vi "elevatorStatesLogic.vi"(9 "oldState":T1, 10 "newState":T1, 11 "timer":i32) -> (0 "State":T1, 1 "manual?":bool, 2 "Numeric":i32, 3 "elevatorActive":bool)   [LabVIEW 2014]
uses:
  ElevatorStates.ctl
  Global Data!!!.vi
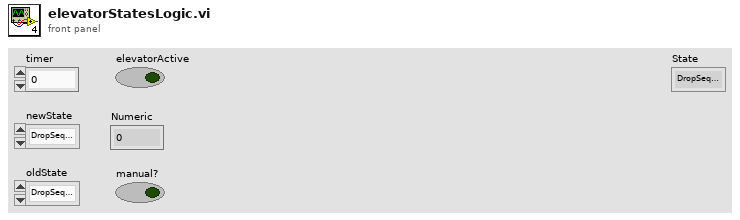
[diagram p1: front panel]
types:
  T1 = typedef "ElevatorStates.ctl" = enum16{"DropSequence", "Reset", "Drop1Stage", "2StageEngage", "Lift1Stage", "1StageEngage", "Rest", "InterruptedLift", "Manual", "Auto2Man", "Initialize", "FeederMode"}
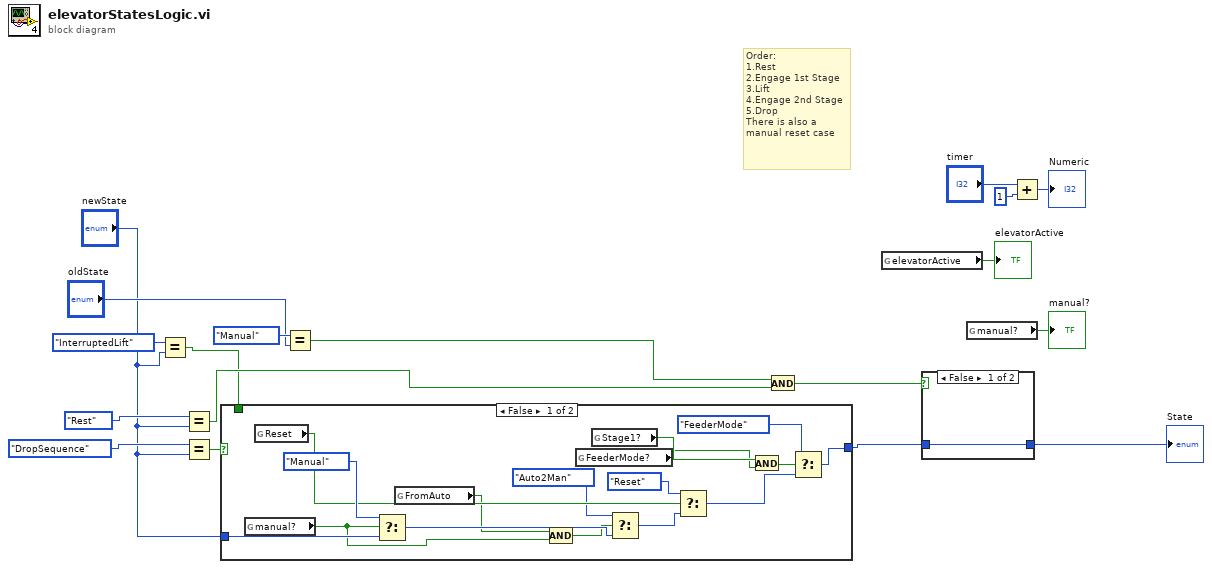
[diagram p0: block diagram]
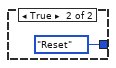
[diagram p2: hidden frame]
diagram:
  # "Order:\n1.Rest\n2.Engage 1st Stage\n3.Lift\n4.Engage 2nd Stage\n5.Drop\nThere is also a \nmanual reset case"
  n1 = Equal?(x=ElevatorStates."InterruptedLift", y="newState") -> (x = y?=w2:bool)
  n2 = Equal?(x=ElevatorStates."Rest", y="newState") -> (x = y?=w7:bool)
  n3 = Equal?(x=ElevatorStates."DropSequence", y="newState") -> (x = y?=w15:bool)
  n4 = case shown="False" w15 {
    tunnel: [w23 w35] -> w6
    tunnel: "newState" -> [w31 w35]
    tunnel: w2 -> [_ _]
    frame False {
      n5 = global read "Global Data!!!.vi" "manual?"() -> (w26:bool)
      n6 = global read "Global Data!!!.vi" "Reset"() -> (w33:bool)
      n7 = Select(t=ElevatorStates."Manual" ("Enum"), s=w26, f=w31) -> (s? t:f=w29:T1)
      n8 = global read "Global Data!!!.vi" "FromAuto"() -> (w25:bool)
      n9 = Compound Arithmetic op=AND(w25, w26) -> (w27:bool)
      n10 = global read "Global Data!!!.vi" "FeederMode?"() -> (w19:bool)
      n11 = global read "Global Data!!!.vi" "Stage1?"() -> (w20:bool)
      n12 = Select(t=ElevatorStates."Auto2Man", s=w27, f=w29) -> (s? t:f=w30:T1)
      n13 = Select(t=ElevatorStates."Reset" ("Enum"), s=w33, f=w30) -> (s? t:f=w24:T1)
      n14 = And(x=w20, y=w19) -> (x .and. y?=w21:bool)
      n15 = Select(t=ElevatorStates."FeederMode", s=w21, f=w24) -> (s? t:f=w23:T1)
    }
    frame True {
    }
  }
  n16 = Equal?(x=ElevatorStates."Manual", y="oldState") -> (x = y?=w9:bool)
  n17 = And(x=w9, y=w7) -> (x .and. y?=w10:bool)
  n18 = global read "Global Data!!!.vi" "elevatorActive"() -> (→"elevatorActive":bool)
  n19 = case shown="False" w10 {
    tunnel: w6 -> [w36 _]
    tunnel: [w36 ElevatorStates."Reset" ("newState")] -> w1
    frame False {
    }
    frame True {
    }
  }
  "State" <- w1
  n20 = global read "Global Data!!!.vi" "manual?"() -> (→"manual?":bool)
  n21 = Add(x="timer", y=1) -> (x+y=→"Numeric":i32)
